vi "AlliGator Install New Version.vi"(8 "Error In":errorcluster, 11 "AlliGator Installer Web Address":string) -> (0 "Error Out":errorcluster, 1 "standard error":string, 2 "standard output":string, 3 "return code":i32)   [LabVIEW 2021, in "AlliGator GUI.lvlib"]
doc: "Installs the latest AlliGator version listed on the ReadTheDocs website."
uses:
  AlliGator GUI.lvlib
  <vilib>/Utility/error.llb/DialogType.ctl
  <userlib>/_OpenG.lib/lvzip/lvzip.llb/subVI/ZLIB Extract All Files To Dir (Path)__ogtk.vi
  <vilib>/zip/NI_Unzip.lvlib
  Files/Files.lvlib
  Error/Error.lvlib
  GUI/GUI.lvlib
panel:
  out "standard output 2":string
  out "standard error 2":string
  out "return code 2":i32
  in  "Message":string
  out "Progress Bar":dbl(slide) scale=0.0..100.0
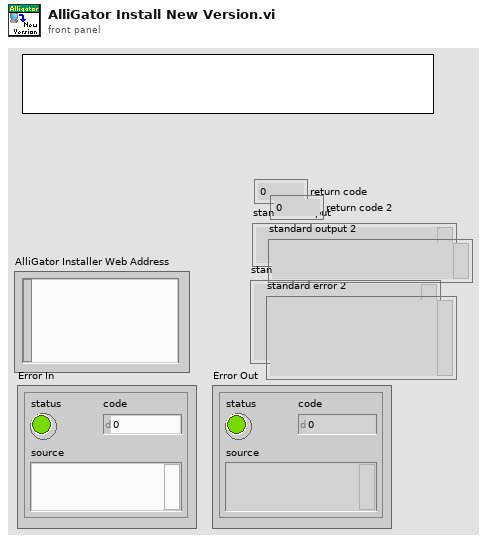
[diagram p1: front panel]
types:
  T1 = typedef "AlliGator Progress Bar Q Element.ctl" = cluster{"Action":string, "Value":dbl}
  T2 = typedef "DialogType.ctl" = u16
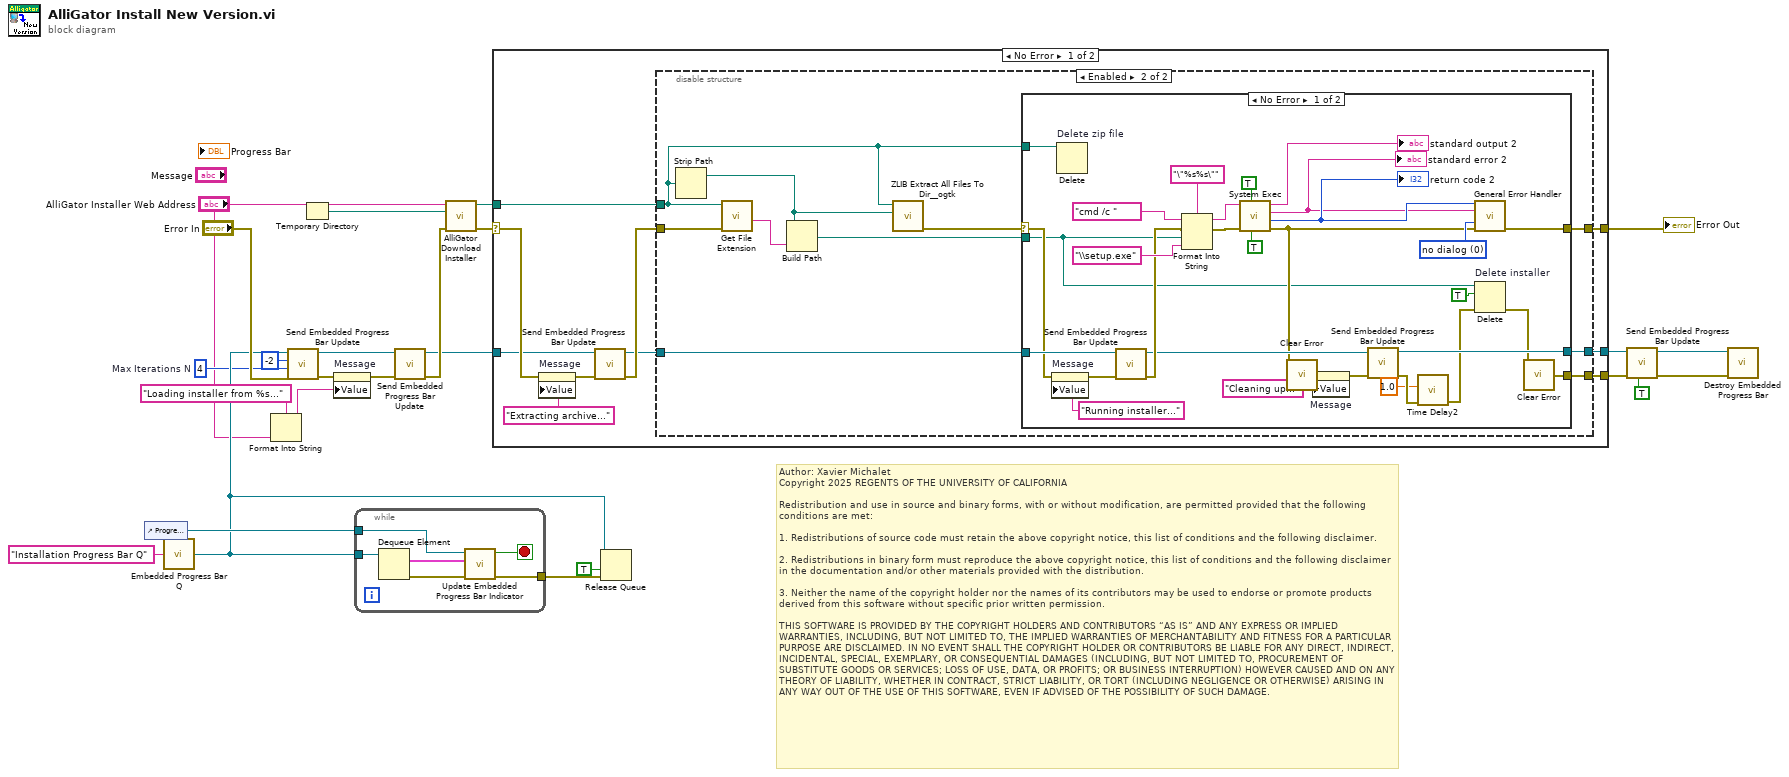
[diagram p0: block diagram]
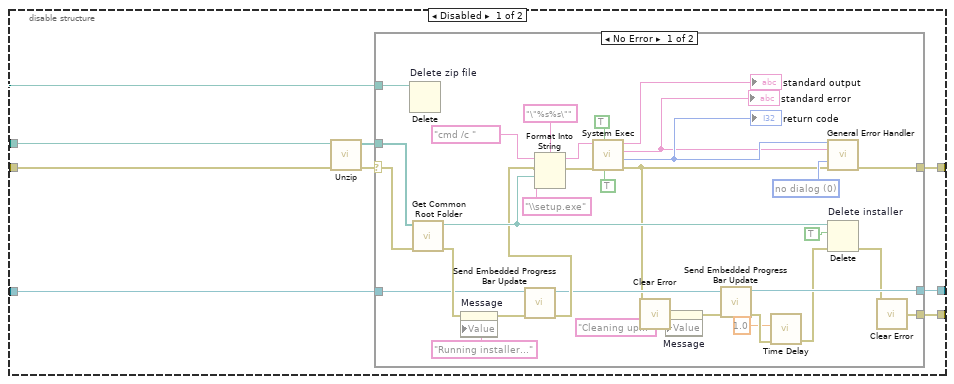
[diagram p2: hidden frame]
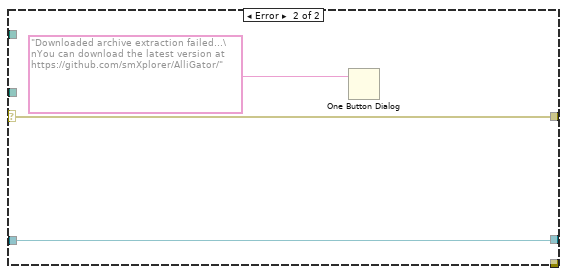
[diagram p3: hidden frame]
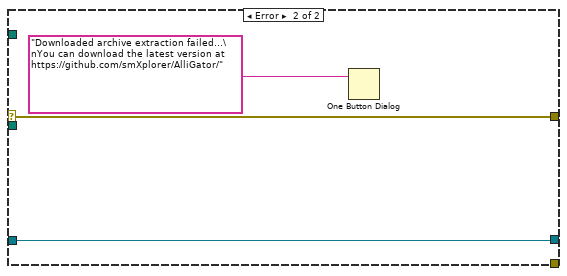
[diagram p4: hidden frame]
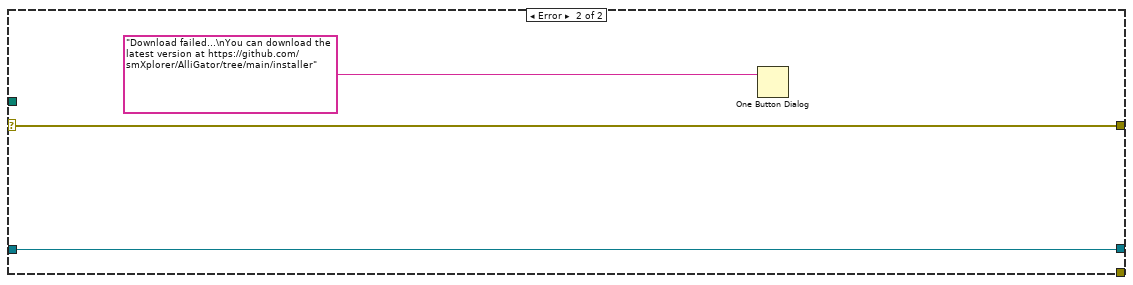
[diagram p5: hidden frame]
diagram:
  w14 = 4  # Max Iterations N
  # "Author: Xavier Michalet\nCopyright 2025 REGENTS OF THE UNIVERSITY OF CALIFORNIA\n\nRedistribution and use in source and binary forms, with or without modification, are permitted provided that the following conditions are met:\n\n1. Redistributions of source code must retain the above copyright notice, this list of conditions and the following disclaimer.\n\n2. Redistributions in binary form must reproduce the above copyright notice, this list of conditions and the following disclaimer in the documentation and/or other materials provided with the distribution.\n\n3. Neither the name of the copyright holder nor the names of its contributors may be used to endorse or promote products derived from this software without specific prior written permission.\n\nTHIS SOFTWARE IS PROVIDED BY THE COPYRIGHT HOLDERS AND CONTRIBUTORS “AS IS” AND ANY EXPRESS OR IMPLIED WARRANTIES, INCLUDING, BUT NOT LIMITED TO, THE IMPLIED WARRANTIES OF MERCHANTABILITY AND FITNESS FOR A PARTICULAR PURPOSE ARE DISCLAIMED. IN NO EVENT SHALL THE COPYRIGHT HOLDER OR CONTRIBUTORS BE LIABLE FOR ANY DIRECT, INDIRECT, INCIDENTAL, SPECIAL, EXEMPLARY, OR CONSEQUENTIAL DAMAGES (INCLUDING, BUT NOT LIMITED TO, PROCUREMENT OF SUBSTITUTE GOODS OR SERVICES; LOSS OF USE, DATA, OR PROFITS; OR BUSINESS INTERRUPTION) HOWEVER CAUSED AND ON ANY THEORY OF LIABILITY, WHETHER IN CONTRACT, STRICT LIABILITY, OR TORT (INCLUDING NEGLIGENCE OR OTHERWISE) ARISING IN ANY WAY OUT OF THE USE OF THIS SOFTWARE, EVEN IF ADVISED OF THE POSSIBILITY OF SUCH DAMAGE."
  n1 = control-ref of="Progress Bar"() -> (w20:refnum<vi>)
  n2 = call "Embedded Progress Bar Q.vi"("Progress Bar Queue Name"="Installation Progress Bar Q") -> ("Progress Bar Queue"=w15:refnum<queue>)  [unwired: 6 in]
  n3 = Format Into String(format string="Loading installer from %s..." ("Message"), "AlliGator Installer Web Address") -> (resulting string=w11:string)  [unwired: 2 in, 1 out]
  n4 = call "Send Embedded Progress Bar Update.vi"("Error In"="Error In", "Max Iterations N"=w14, "Current Iteration i (i or -1: standard or || iteration; 0 or -2: first standard or || iteration)"=-2 ("Current Iteration i (-1: || iteration, -2: first || iteration)"), "Progress Bar Queue in"=w15) -> ("Error Out"=w13:errorcluster, "Progress Bar Queue out"=w9:refnum<queue>)  [unwired: 6 in]
  n5 = Temporary Directory() -> (w22:path)
  n6 = property on="Message" class="Str"(error in=w13, "Value"=w11) -> (error out=w8:errorcluster)  [unwired: 1 in, 1 out]
  n7 = while {
    tunnel: w15 -> [w31]
    tunnel: w20 -> [w29]
    tunnel: [w26] -> w19
    stop <- w27 stop-if-true
    n8 = Dequeue Element(queue=w31) -> (element=w30:T1, error out=w28:errorcluster)  [unwired: 2 in, 2 out]
    n9 = call "Update Embedded Progress Bar Indicator.vi"("Error In"=w28, "Progress Bar Event"=w30, "Progress Bar Refnum"=w29) -> ("Error Out"=w26:errorcluster, "Quit?"=w27:bool)  [unwired: 7 in]
  }
  n10 = call "Send Embedded Progress Bar Update.vi"("Error In"=w8, "Progress Bar Queue in"=w9) -> ("Error Out"=w7:errorcluster, "Progress Bar Queue out"=w6:refnum<queue>)  [unwired: 8 in]
  n11 = call "AlliGator Download Installer.vi"("Error In"=w7, "Dest Folder"=w22, "URL"="AlliGator Installer Web Address") -> ("Error Out"=w24:errorcluster, "File Path"=w23:path)  [unwired: 5 in, 2 out]
  n12 = case shown="No Error" w24 {
    selector: w24 -> [w39 w131]
    tunnel: [w40 w131] -> w25
    tunnel: w23 -> [w41 _]
    tunnel: w6 -> [w37 w130]
    tunnel: [w33 w130] -> w3
    tunnel: [w32 _] -> w2
    frame No Error {
      n13 = property on="Message" class="Str"(error in=w39, "Value"="Extracting archive..." ("Message")) -> (error out=w38:errorcluster)  [unwired: 1 in, 1 out]
      n14 = call "Send Embedded Progress Bar Update.vi"("Error In"=w38, "Progress Bar Queue in"=w37) -> ("Error Out"=w35:errorcluster, "Progress Bar Queue out"=w34:refnum<queue>)  [unwired: 8 in]
      n15 = disable-structure shown="Enabled" {
        disable-tunnel: w41 -> [w49 w90]
        disable-tunnel: [w46 w95] -> w40
        disable-tunnel: w35 -> [w45 w89]
        disable-tunnel: w34 -> [w44 w94]
        disable-tunnel: [w43 w93] -> w33
        disable-tunnel: [w42 w92] -> w32
        frame Disabled {
          n16 = call <vilib>:"Unzip.vi"("error in (no error)"=w45, "Zip file"=w49) -> ("error out"=w48:errorcluster, "Unzipped files"=w47:path[])  [unwired: 7 in, 1 out]
          n17 = case shown="No Error" w48 {
            selector: w48 -> [w71 w83]
            tunnel: [w70 w83] -> w46
            tunnel: w49 -> [w82 _]
            tunnel: w47 -> [w75 _]
            tunnel: w44 -> [w62 w84]
            tunnel: [w54 w84] -> w43
            tunnel: [w52 _] -> w42
            frame No Error {
              w67 = T2 0 items=["no dialog", "OK message", "continue or stop message", "OK message + warnings", "continue/stop + warnings"] ("type of dialog (OK msg:1)")
              n18 = Delete "Delete zip file"(path (use dialog)=w82) -> ()  [unwired: 4 in, 3 out]
              n19 = call "Get Common Root Folder.vi"("Error In"=w71, "Array of File Paths"=w75) -> ("Error Out"=w65:errorcluster, "Common Folder Path"=w74:path)  [unwired: 8 in]
              n20 = property on="Message" class="Str"(error in=w65, "Value"="Running installer..." ("Message")) -> (error out=w63:errorcluster)  [unwired: 1 in, 1 out]
              n21 = call "Send Embedded Progress Bar Update.vi"("Error In"=w63, "Progress Bar Queue in"=w62) -> ("Error Out"=w61:errorcluster, "Progress Bar Queue out"=w58:refnum<queue>)  [unwired: 8 in]
              n22 = Format Into String(format string="\"%s%s\"" ("command line"), initial string="cmd /c ", error in=w61, w74, "\\setup.exe") -> (resulting string=w80:string, error out=w81:errorcluster)
              n23 = call <vilib>:"System Exec.vi"("run minimized? (F)"=TRUE, "wait until completion? (T)"=TRUE, "error in (no error)"=w81, "command line"=w80) -> ("error out"=w57:errorcluster, "return code"=w69:i32, "standard error"=w68:string, "standard output"=→"standard output":string)  [unwired: 4 in]
              "standard error" <- w68
              "return code" <- w69
              n24 = call "Clear Error.vi"("Error In"=w57) -> ("no Error Out"=w55:errorcluster)  [unwired: 8 in]
              n25 = property on="Message" class="Str"(error in=w55, "Value"="Cleaning up..." ("Message")) -> (error out=w59:errorcluster)  [unwired: 1 in, 1 out]
              n26 = call "Send Embedded Progress Bar Update.vi"("Error In"=w59, "Progress Bar Queue in"=w58) -> ("Error Out"=w56:errorcluster, "Progress Bar Queue out"=w54:refnum<queue>)  [unwired: 8 in]
              n27 = call "Time Delay"("error in (no error)"=w56, "Delay Time (s)"=1.0) -> ("error out"=w51:errorcluster)  [unwired: 9 in]
              n28 = call <vilib>:"General Error Handler.vi"("[error code] (0)"=w69, "[error source] (\" \")"=w68, "type of dialog (OK msg:1)"=w67, "error in (no error)"=w57) -> ("error out"=w70:errorcluster)  [unwired: 7 in, 4 out]
              n29 = Delete "Delete installer"(path (use dialog)=w74, entire hierarchy (F)=TRUE, error in=w51) -> (error out=w53:errorcluster)  [unwired: 2 in, 2 out]
              n30 = call "Clear Error.vi"("Error In"=w53) -> ("no Error Out"=w52:errorcluster)  [unwired: 8 in]
            }
            frame Error {
              n31 = One Button Dialog(message="Downloaded archive extraction failed...\nYou can download the latest version at https://github.com/smXplorer/AlliGator/") -> ()  [unwired: 1 in, 1 out]
            }
          }
        }
        frame Enabled {
          n32 = Strip Path(path=w90) -> (stripped path=w87:path)  [unwired: 1 out]
          n33 = call <vilib>:"Get File Extension.vi"("error in (no error)"=w89, "file"=w90) -> ("filename without extension"=w88:string)  [unwired: 5 in, 4 out]
          n34 = Build Path(base path=w87, name or relative path=w88) -> (appended path=w86:path)
          n35 = call-poly <userlib>:"ZLIB Extract All Files To Dir__ogtk.vi"("destination directory (archive name without ending)"=w87, "archive name (file dialog)"=w90) -> ("error out"=w91:errorcluster)  [unwired: 7 in, 2 out]
          n36 = case shown="No Error" w91 {
            selector: w91 -> [w97 w127]
            tunnel: [w117 w127] -> w95
            tunnel: w90 -> [w126 _]
            tunnel: w94 -> [w110 w128]
            tunnel: [w102 w128] -> w93
            tunnel: [w100 _] -> w92
            tunnel: w86 -> [w96 _]
            frame No Error {
              w114 = T2 0 items=["no dialog", "OK message", "continue or stop message", "OK message + warnings", "continue/stop + warnings"] ("type of dialog (OK msg:1)")
              n37 = property on="Message" class="Str"(error in=w97, "Value"="Running installer..." ("Message")) -> (error out=w111:errorcluster)  [unwired: 1 in, 1 out]
              n38 = Delete "Delete zip file"(path (use dialog)=w126) -> ()  [unwired: 4 in, 3 out]
              n39 = call "Send Embedded Progress Bar Update.vi"("Error In"=w111, "Progress Bar Queue in"=w110) -> ("Error Out"=w109:errorcluster, "Progress Bar Queue out"=w106:refnum<queue>)  [unwired: 8 in]
              n40 = Format Into String(format string="\"%s%s\"" ("command line"), initial string="cmd /c ", error in=w109, w96, "\\setup.exe") -> (resulting string=w124:string, error out=w125:errorcluster)
              n41 = call <vilib>:"System Exec.vi"("run minimized? (F)"=TRUE, "wait until completion? (T)"=TRUE, "error in (no error)"=w125, "command line"=w124) -> ("error out"=w105:errorcluster, "return code"=w116:i32, "standard error"=w115:string, "standard output"=→"standard output 2":string)  [unwired: 4 in]
              "standard error 2" <- w115
              "return code 2" <- w116
              n42 = call "Clear Error.vi"("Error In"=w105) -> ("no Error Out"=w103:errorcluster)  [unwired: 8 in]
              n43 = property on="Message" class="Str"(error in=w103, "Value"="Cleaning up..." ("Message")) -> (error out=w107:errorcluster)  [unwired: 1 in, 1 out]
              n44 = call "Send Embedded Progress Bar Update.vi"("Error In"=w107, "Progress Bar Queue in"=w106) -> ("Error Out"=w104:errorcluster, "Progress Bar Queue out"=w102:refnum<queue>)  [unwired: 8 in]
              n45 = call "Time Delay2"("error in (no error)"=w104, "Delay Time (s)"=1.0) -> ("error out"=w99:errorcluster)  [unwired: 9 in]
              n46 = call <vilib>:"General Error Handler.vi"("[error code] (0)"=w116, "[error source] (\" \")"=w115, "type of dialog (OK msg:1)"=w114, "error in (no error)"=w105) -> ("error out"=w117:errorcluster)  [unwired: 7 in, 4 out]
              n47 = Delete "Delete installer"(path (use dialog)=w96, entire hierarchy (F)=TRUE, error in=w99) -> (error out=w101:errorcluster)  [unwired: 2 in, 2 out]
              n48 = call "Clear Error.vi"("Error In"=w101) -> ("no Error Out"=w100:errorcluster)  [unwired: 8 in]
            }
            frame Error {
              n49 = One Button Dialog(message="Downloaded archive extraction failed...\nYou can download the latest version at https://github.com/smXplorer/AlliGator/") -> ()  [unwired: 1 in, 1 out]
            }
          }
        }
      }
    }
    frame Error {
      n50 = One Button Dialog(message="Download failed...\nYou can download the latest version at https://github.com/smXplorer/AlliGator/tree/main/installer") -> ()  [unwired: 1 in, 1 out]
    }
  }
  "Error Out" <- w25
  n51 = Release Queue(queue=w15, force destroy? (F)=TRUE, error in (no error)=w19) -> ()  [unwired: 3 out]
  n52 = call "Send Embedded Progress Bar Update.vi"("Stop Progress Bar (F)"=TRUE, "Error In"=w2, "Progress Bar Queue in"=w3) -> ("Error Out"=w4:errorcluster, "Progress Bar Queue out"=w5:refnum<queue>)  [unwired: 7 in]
  n53 = call "Destroy Embedded Progress Bar.vi"("Error In"=w4, "Progress Bar Queue in"=w5) -> ()  [unwired: 9 in, 1 out]
